vi "CM-Init Slot Controls.vi"(0 "slot ctl refs":refnum<vi>[](array[refnum]), 5 "Devices":T1[](array[typedef]), 9 "config file":path, 11 "error in (no error)":errorcluster) -> (4 "slot ctl refs out":refnum<vi>[](array[refnum]), 6 "Devices thru":T1[](array[typedef]), 15 "error out":errorcluster)   [LabVIEW 2020]
uses:
  Type Defs/General PXISlot XControl/PXISlotGP.xctl
  PXI DAQ VIs/Type Defs/PXI-Device Spec.ctl
  Type Defs/PXISlot XControl/Connector Type.ctl
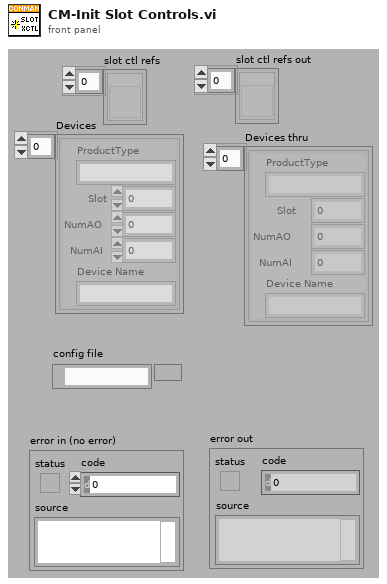
[diagram p1: front panel]
types:
  T1 = typedef "PXI-Device Spec.ctl" = cluster{"Slot":i32, "ProductType":string, "NumAO":i32, "NumAI":i32, "Device Name":string}
  T2 = typedef "Connector Type.ctl" = enum16{"None", "PXI-4461", "BNC-2110", "BNC-2090", "PXIe-4463", "PXIe-4464"}
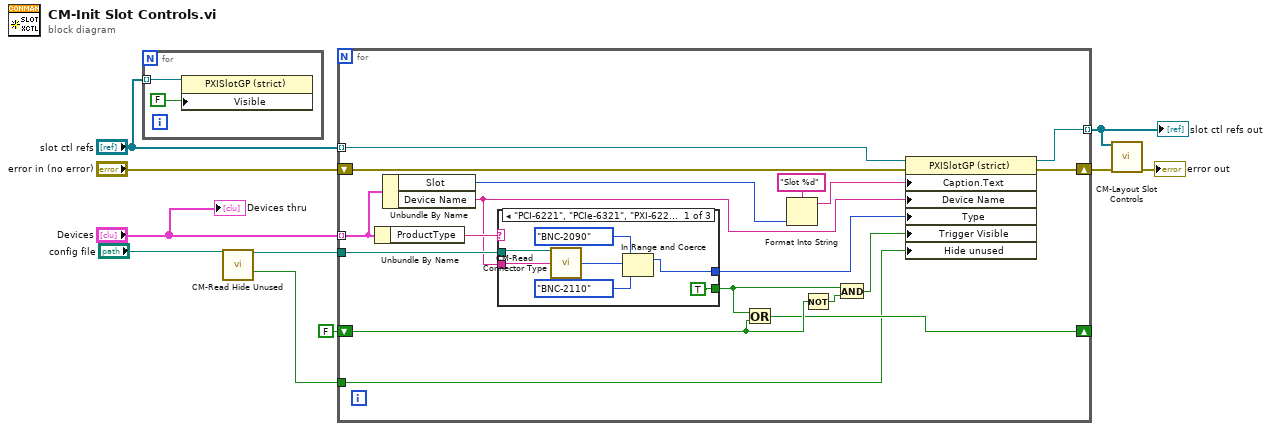
[diagram p0: block diagram]
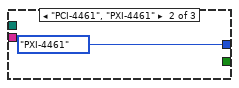
[diagram p2: hidden frame]
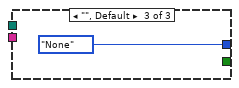
[diagram p3: hidden frame]
diagram:
  n1 = for {
    tunnel: "slot ctl refs" -> [w12] mode=indexing
    n2 = property class="PXISlotGP (strict)"(reference=w12, "Visible"=FALSE) -> ()  [unwired: 1 in, 2 out]
  }
  n3 = call "CM-Read Hide Unused.vi"("configuration file path"="config file") -> ("file path"=w1:path, "Hide unused"=w2:bool)  [unwired: 12 in, 1 out]
  n4 = for {
    tunnel: "slot ctl refs" -> [w28] mode=indexing
    shift-right: [w29] -> w6
    shift-left: "error in (no error)" -> [w30]
    tunnel: "Devices" -> [w24] mode=indexing
    shift-right: [w22] -> _
    shift-left: FALSE -> [w23]
    tunnel: [w20] -> w4 mode=indexing
    tunnel: w2 -> [w15]
    tunnel: w1 -> [w14]
    n5 = Unbundle By Name(w24) -> ("ProductType"=w27:string)
    n6 = Unbundle By Name(w24) -> ("Slot"=w21:i32, "Device Name"=w13:string)
    n7 = case shown="\"PCI-6221\", \"PCIe-6321\", \"PXI-6221\", \"PXIe-6341\", \"USB-6002\", \"USB-6221 (BNC)\", \"USB-6341 (BNC)\"" w27 {
      tunnel: [w31 Connector_Type."PXI-4461" ("Connector Type") Connector_Type."None" ("Connector Type")] -> w26
      tunnel: [TRUE _ _] -> w25
      tunnel: w14 -> [w36 _ _]
      tunnel: w13 -> [w35 _ _]
      frame "PCI-6221", "PCIe-6321", "PXI-6221", "PXIe-6341", "USB-6002", "USB-6221 (BNC)", "USB-6341 (BNC)" {
        n8 = call "CM-Read Connector Type.vi"("configuration file path"=w36, "Device"=w35) -> ("Connector Type"=w34:T2)  [unwired: 11 in, 2 out]
        n9 = In Range and Coerce(upper limit=Connector_Type."BNC-2090", x=w34, lower limit=Connector_Type."BNC-2110") -> (coerced(x)=w31:T2)  [unwired: 1 out]
      }
      frame "PCI-4461", "PXI-4461" {
      }
      frame "", Default {
      }
    }
    n10 = Or(x=w25, y=w23) -> (x .or. y?=w22:bool)
    n11 = Format Into String(format string="Slot %d", w21) -> (resulting string=w16:string)  [unwired: 2 in, 1 out]
    n12 = Not(x=w23) -> (.not. x?=w19:bool)
    n13 = And(x=w25, y=w19) -> (x .and. y?=w18:bool)
    n14 = property class="PXISlotGP (strict)"(reference=w28, error in=w30, "Caption.Text"=w16, "Device Name"=w13, "Type"=w26, "Trigger Visible"=w18, "Hide unused"=w15) -> (reference out=w20:refnum<vi>, error out=w29:errorcluster)
  }
  "slot ctl refs out" <- w4
  n15 = call "CM-Layout Slot Controls.vi"("SlotRefs"=w4, "error in (no error)"=w6) -> ("error out"=→"error out":errorcluster)  [unwired: 13 in]
  "Devices thru" <- "Devices"
